vi "file_LabVIEW_4a.vi"() -> ()   [LabVIEW 2015]
uses:
  <vilib>/Instr/_visa.llb/VISA Configure Serial Port (Instr).vi
panel:
  out "SETPOINT & \nOUTPUT POSISI":cluster{i16, i16}(knob)={0, 102} scale=0.0..360.0
  in  "SETPOINT":i16(knob) scale=0.0..360.0
  out "Grafik Encoder":cluster{"Dial":i16, "y":dbl}(graph)
  out "read buffer":string
  out "PWM":i16(slide) scale=-255.0..255.0
  in  "VISA resource name":refnum<visa-resource-name>
  in  "stop":bool
  out "Grafik PWM":i32(graph)
  # "KONTROL POSISI POROS"
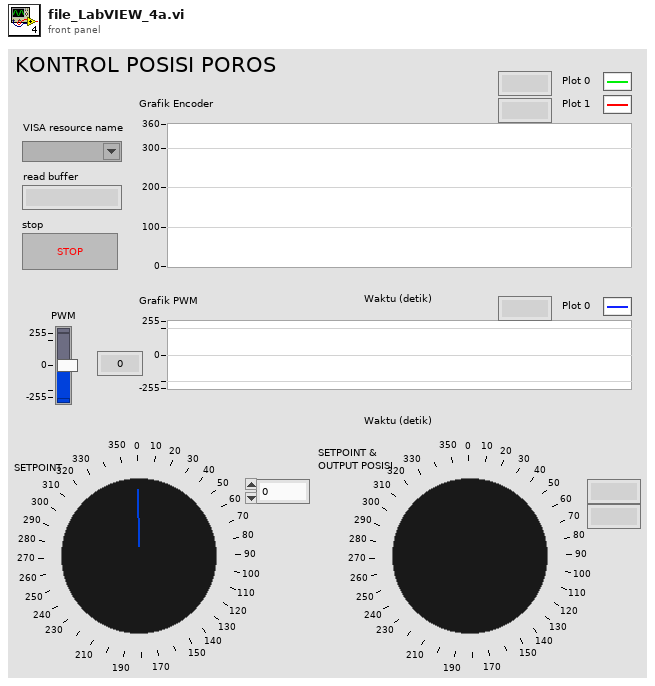
[diagram p1: front panel]
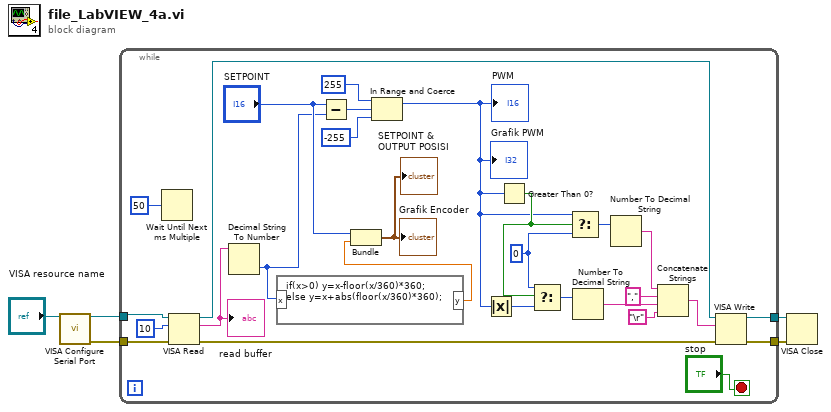
[diagram p0: block diagram]
diagram:
  n1 = call-poly "VISA Configure Serial Port"("VISA resource name"="VISA resource name") -> ("VISA resource name out"=w3:refnum<visa-resource-name>, "error out"=w2:errorcluster)  [unwired: 13 in]
  n2 = while {
    tunnel: [w33] -> w5
    tunnel: [w32] -> w4
    tunnel: w3 -> [w20]
    tunnel: w2 -> [w21]
    stop <- "stop" stop-if-true
    w31 = 0
    n3 = Wait Until Next ms Multiple(millisecond multiple=u32 50) -> ()  [unwired: 1 out]
    n4 = VISA Read(VISA resource name=w20, byte count=u32 10, error in (no error)=w21) -> (VISA resource name out=w6:refnum<visa-resource-name>, read buffer=w16:string, error out=w19:errorcluster)  [unwired: 1 out]
    "read buffer" <- w16
    n5 = Decimal String To Number(string=w16) -> (number=w8:i32)  [unwired: 2 in, 1 out]
    n6 = formula code="if(x>0) y=x-floor(x/360)*360;\nelse y=x+abs(floor(x/360)*360);"("x"=w8) -> ("y"=w7:dbl)
    n7 = Subtract(x="SETPOINT", y=w8) -> (x-y=w12:i32)
    n8 = Bundle "Bundle"("SETPOINT"="SETPOINT", "y"=w7) -> (→"Grafik Encoder" →"SETPOINT & \nOUTPUT POSISI":cluster{"SETPOINT":i16, "y":dbl})  [unwired: 1 in]
    n9 = In Range and Coerce(upper limit=255, x=w12, lower limit=-255) -> (coerced(x)=w9:i32)  [unwired: 1 out]
    "Grafik PWM" <- w9
    "PWM" <- w9
    n10 = Absolute Value(x=w9) -> (abs(x)=w30:i32)
    n11 = Greater Than 0?(x=w9) -> (x > 0?=w15:bool)
    n12 = Select(t=w31, s=w15, f=w30) -> (s? t:f=w28:i32)
    n13 = Select(t=w9, s=w15, f=w31) -> (s? t:f=w29:i32)
    n14 = Number To Decimal String(number=w28) -> (decimal integer string=w25:string)  [unwired: 1 in]
    n15 = Number To Decimal String(number=w29) -> (decimal integer string=w27:string)  [unwired: 1 in]
    n16 = Concatenate Strings "Concatenate Strings"(w27, "," ("string"), w25, "\r") -> (w24:string)
    n17 = VISA Write(VISA resource name=w6, write buffer=w24, error in (no error)=w19) -> (VISA resource name out=w32:refnum<visa-resource-name>, error out=w33:errorcluster)  [unwired: 1 out]
  }
  n18 = VISA Close(VISA resource name=w4, error in (no error)=w5) -> ()  [unwired: 1 out]
